vi "PS35_JoyFEx.vi"(0 "Axis number":i32=1 min=1 max=3, 1 "Control unit ID":i32=1 min=1 max=10, 2 "dValue-In":dbl format="%.3f", 3 "error in (no error)":errorcluster, 5 "function":bool) -> (7 "dValue-Out":dbl format="%.3f", 9 "error out":errorcluster)   [LabVIEW 2020]
doc: "PS35_JoyFEx.vi, created: 06.03.2009 alex; last change: 22.10.2019 alex;\n\n<B>FUNCTIONS:</B> \n\n<B>Read:</B> FALSE: read maximum velocity of an axis \nfor joystick mode (values in selected unit).\n<B>Write:</B> TRUE: set maximum velocity of an axis \nfor joystick mode (values in selected unit).\nThe maximum speed for the full joystick excursion will be defined with\nthis function. The sign defines the positioning direction of the joystick.\nvelocity = unit/s\n----------------------------------------------------------------------------------------\n<B>INPUT:</B>\n[TF] <B>function:</B> function selector. (Read, Write)\n[I32] <B>Control unit ID:</B> control unit index. (Default=1, Range=1...10)\n[I32] <B>Axis number:</B> axis number. (Default=1, Range=1...3)\n[DBL] <B>dValue-In:</B> velocity value. (only for Write: Default=0.0)\n[CLU] <B>error in</B>\n----------------------------------------------------------------------------------------\n<B>OUTPUT:</B>\n[DBL] <B>dValue-Out:</B> velocity value. (for Write: dValue-Out=dValue-In)\n[CLU] <B>error out</B>\n----------------------------------------------------------------------------------------\n<B>SUB-VIs:</B>\nPS35_GetReadError.vi\n----------------------------------------------------------------------------------------\n<B>EXT-Calls:</B>\nps35.dll (V2.01)\n----------------------------------------------------------------------------------------"
uses:
  ps35.dll
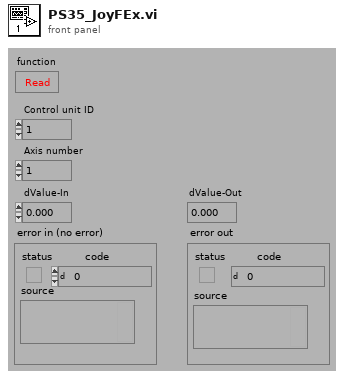
[diagram p1: front panel]
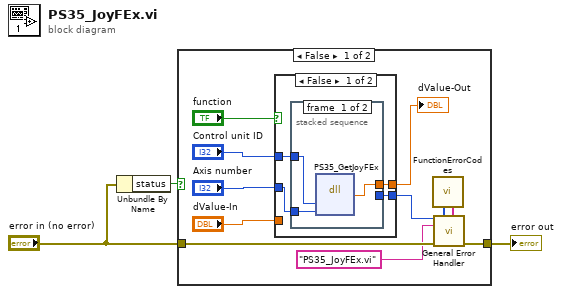
[diagram p0: block diagram]
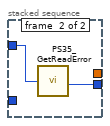
[diagram p2: hidden frame]
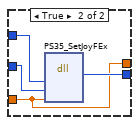
[diagram p3: hidden frame]
diagram:
  n1 = Unbundle By Name("error in (no error)") -> ("status"=w1:bool)
  n2 = case shown="False" w1 {
    tunnel: "error in (no error)" -> [w14 w28]
    tunnel: [w13 w28] -> w3
    frame False {
      n3 = case shown="False" "function" {
        tunnel: "Control unit ID" -> [w17 w26]
        tunnel: [w18 w27] -> w10
        tunnel: "dValue-In" -> [_ w24]
        tunnel: [w16 w24] -> w8
        tunnel: "Axis number" -> [w15 w25]
        frame False {
          n4 = stacked-sequence {
            tunnel: [_ w23] -> w18
            tunnel: w17 -> [w21 w22]
            tunnel: [w20 _] -> w16
            tunnel: w15 -> [w19 _]
            frame #0 {
              n5 = dll-call lib="C:/GEECS/Developers Version/source/Device Drivers/OwiSoft/OWISoftOEM/ps35/labview/lv82/ps35.dll" fn="PS35_GetJoyFEx" label="PS35_\nGet\nJoyFEx"("Index"=w21, "AxisNr"=w19) -> ("Rückgabetyp"=w20:dbl)  [unwired: 5 in, 2 out]
            }
            frame #1 {
              n6 = call "PS35_GetReadError.vi"("Control unit ID"=w22) -> ("Read error"=w23:i32)
            }
          }
        }
        frame True {
          n7 = dll-call lib="C:/GEECS/Developers Version/source/Device Drivers/OwiSoft/OWISoftOEM/ps35/labview/lv82/ps35.dll" fn="PS35_SetJoyFEx" label="PS35_\nSet\nJoyFEx"("Index"=w26, "AxisNr"=w25, "dValue"=w24) -> ("Rückgabetyp"=w27:i32)  [unwired: 6 in, 2 out]
        }
      }
      "dValue-Out" <- w8
      n8 = call "FunctionErrorCodes.vi"() -> ("[user-defined codes]"=w4:i32[], "[user-defined descriptions]"=w5:string[])  [unwired: 8 in]
      n9 = call <vilib>:"General Error Handler.vi"("[error code] (0)"=w10, "[user-defined codes]"=w4, "[user-defined descriptions]"=w5, "[error source] (\" \")"="PS35_JoyFEx.vi" ("[error source] (\" \")"), "error in (no error)"=w14) -> ("error out"=w13:errorcluster)  [unwired: 6 in, 4 out]
    }
    frame True {
    }
  }
  "error out" <- w3
